vi "OMR_Automatic_Report_Generation .vi"() -> ()   [LabVIEW 2011]
uses:
  <vilib>/Utility/file.llb/Write To Spreadsheet File (string).vi
  <vilib>/vision/NI_Vision_Development_Module.lvlib
panel:
  out "Result":string[](array[string])
  in  "?":bool
  in  "Tab Control":T1(tab)
  out "Score":dbl
  out "Image 2":T2(plugin-control)
  in  "File Path":path
  out "File Path 2":string
  in  "Marks for\nCorrect Answe":dbl format="%#_6p"
  in  "6 to 10":string[](array[string])
  in  "1 to 5":string[](array[string])
  in  "16 to  20":string[](array[string])
  in  "11 to 15":string[](array[string])
  out "Score 2":dbl format="%_4f"
  out "0 to 5":dbl[](array[numeric])
  out "0 to 6":dbl[](array[numeric])
  out "0 to 7":dbl[](array[numeric])
  out "0 to 8":dbl[](array[numeric])
  out "Centroid (16 to 20)":cluster{"X Centroid":sgl, "Y Centroid":sgl} {"Y Centroid" format="%.2f"; "X Centroid" format="%.2f"}
  out "Centroid (1 to 5)":cluster{"X Centroid":sgl, "Y Centroid":sgl} {"Y Centroid" format="%.2f"; "X Centroid" format="%.2f"}
  out "Centroid (11 to 15)":cluster{"X Centroid":sgl, "Y Centroid":sgl} {"Y Centroid" format="%.2f"; "X Centroid" format="%.2f"}
  out "Centroid (6 to 10)":cluster{"X Centroid":sgl, "Y Centroid":sgl} {"Y Centroid" format="%.2f"; "X Centroid" format="%.2f"}
  out "1 to 5":string[](array[string])
  out "5 to 10":string[](array[string])
  out "11 to 15":string[](array[string])
  out "16 to 20":string[](array[string])
  out "1 to 6":dbl[](array[numeric])
  out "6 to 10":dbl[](array[numeric])
  out "11 to 16":dbl[](array[numeric])
  out "16 to 21":dbl[](array[numeric])
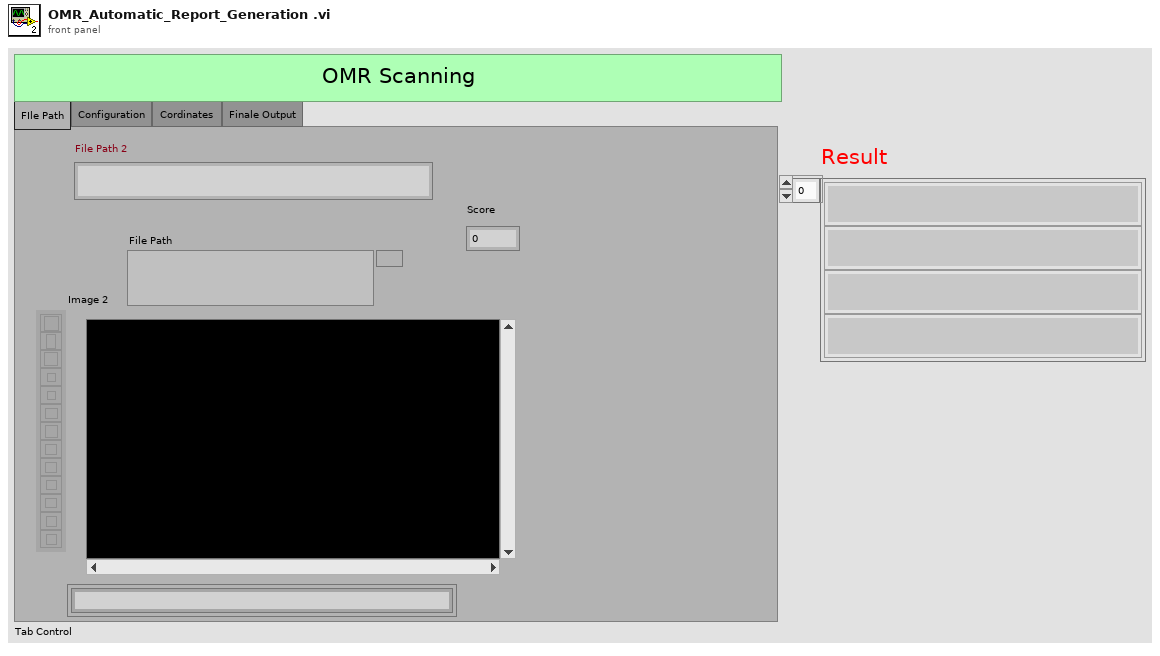
[diagram p1: front panel]
types:
  T1 = enum32{"FIle Path", "Configuration", "Cordinates ", "Finale Output"}
  T2 = typedef "IMAQ Image.ctl" = refnum<image>
  T3 = typedef "Image Type" = u32
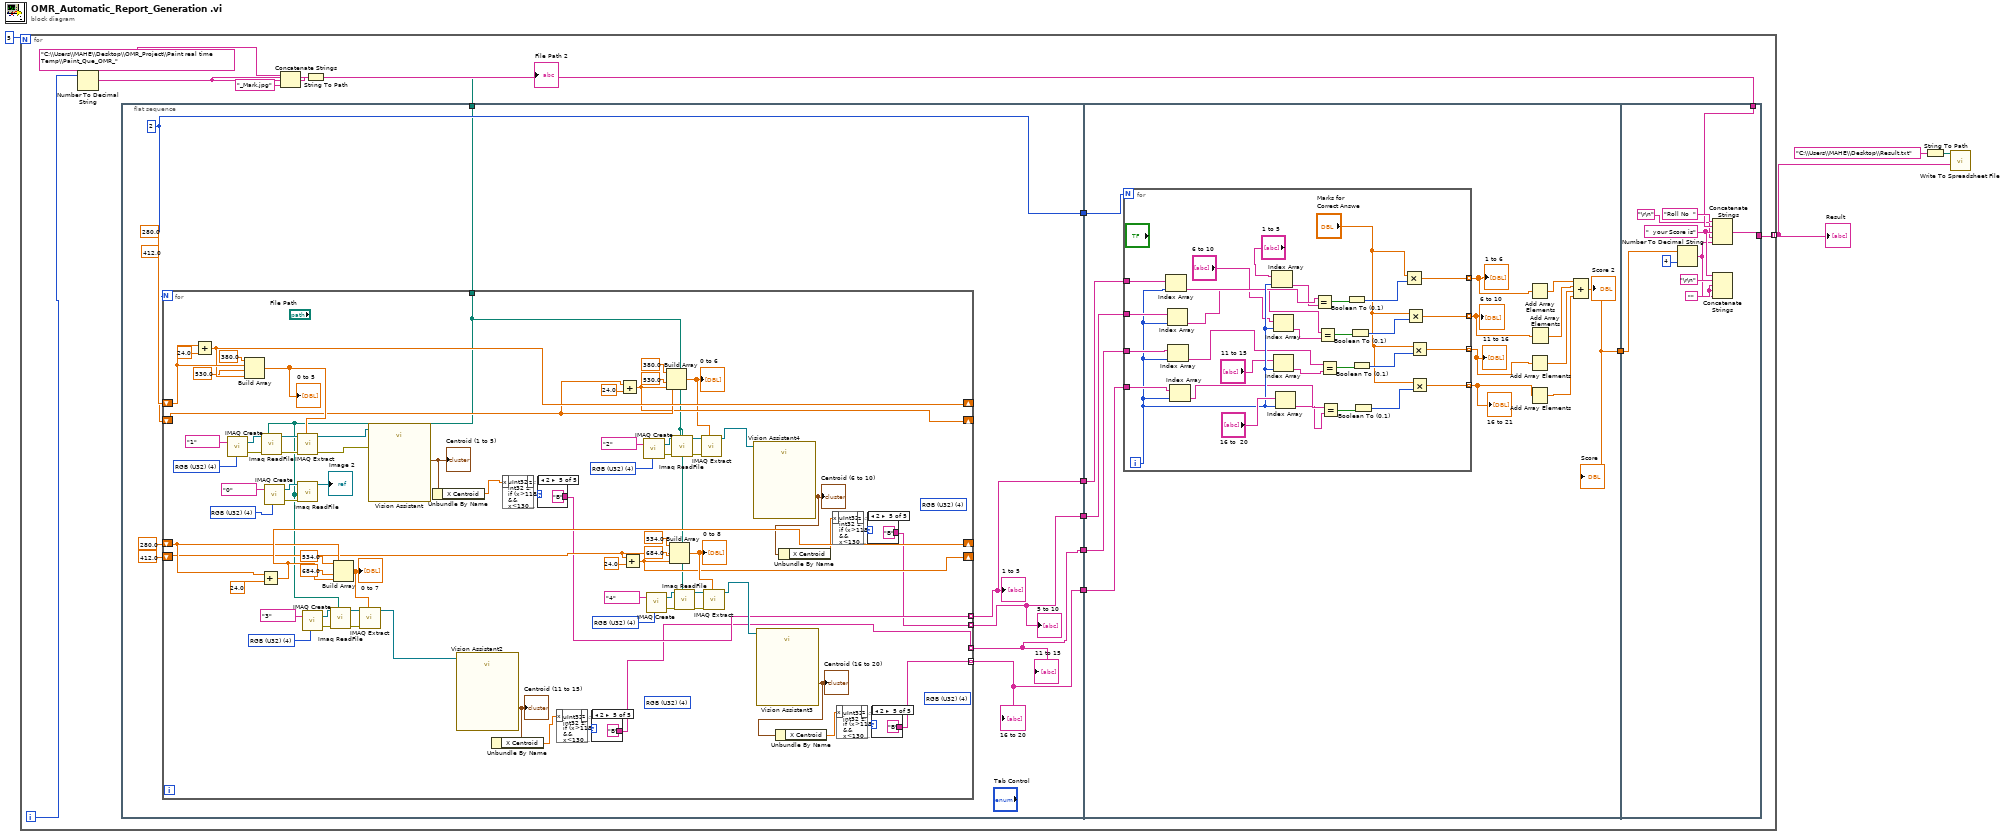
[diagram p0: block diagram]
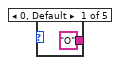
[diagram p2: hidden frame]
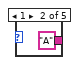
[diagram p3: hidden frame]
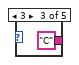
[diagram p4: hidden frame]
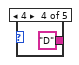
[diagram p5: hidden frame]
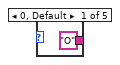
[diagram p6: hidden frame]
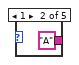
[diagram p7: hidden frame]
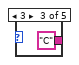
[diagram p8: hidden frame]
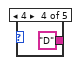
[diagram p9: hidden frame]
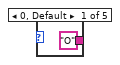
[diagram p10: hidden frame]
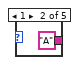
[diagram p11: hidden frame]
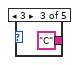
[diagram p12: hidden frame]
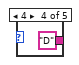
[diagram p13: hidden frame]
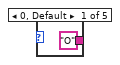
[diagram p14: hidden frame]
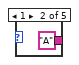
[diagram p15: hidden frame]
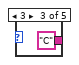
[diagram p16: hidden frame]
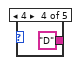
[diagram p17: hidden frame]
diagram:
  n1 = for {
    N: 5 -> [_]
    tunnel: [w5] -> w1 mode=indexing
    i -> [w9]
    n2 = Number To Decimal String(number=w9) -> (decimal integer string=w6:string)  [unwired: 1 in]
    n3 = flat-sequence {
      tunnel: [w23] -> w17
      tunnel: [w21] -> w16
      tunnel: [w22] -> w15
      tunnel: [w19] -> w14
      tunnel: [w20] -> w13
      tunnel: w8 -> [w18]
      tunnel: w17 -> [w135]
      tunnel: w16 -> [w134]
      tunnel: w15 -> [w132]
      tunnel: w14 -> [w133]
      tunnel: w13 -> [w136]
      tunnel: [w123] -> w12
      tunnel: w12 -> [w176]
      tunnel: w6 -> [w171]
      tunnel: [w167] -> w5
      frame #0 {
        w20 = 2
        n4 = for {
          N: w20 -> [_]
          shift-right: [w97] -> _
          shift-left: 280.0 -> [w98]
          shift-right: [w74] -> _
          shift-left: 412.0 -> [w75]
          shift-right: [w52] -> _
          shift-left: 280.0 -> [w50]
          shift-right: [w51] -> _
          shift-left: 412.0 -> [w49]
          tunnel: [w32] -> w23 mode=indexing
          tunnel: [w31] -> w21 mode=indexing
          tunnel: [w30] -> w19 mode=indexing
          tunnel: [w29] -> w22 mode=indexing
          tunnel: w18 -> [w28]
          (unwired) T3 4 items=["Grayscale (U8)", "Grayscale (I16)", "Grayscale (SGL)", "Complex (CSG)", "RGB (U32)", "HSL (U32)", "RGB (U64)"] ("Image Type")
          (unwired) T3 4 items=["Grayscale (U8)", "Grayscale (I16)", "Grayscale (SGL)", "Complex (CSG)", "RGB (U32)", "HSL (U32)", "RGB (U64)"] ("Image Type")
          (unwired) T3 4 items=["Grayscale (U8)", "Grayscale (I16)", "Grayscale (SGL)", "Complex (CSG)", "RGB (U32)", "HSL (U32)", "RGB (U64)"] ("Image Type")
          w59 = T3 4 items=["Grayscale (U8)", "Grayscale (I16)", "Grayscale (SGL)", "Complex (CSG)", "RGB (U32)", "HSL (U32)", "RGB (U64)"] ("Image Type")
          w66 = T3 4 items=["Grayscale (U8)", "Grayscale (I16)", "Grayscale (SGL)", "Complex (CSG)", "RGB (U32)", "HSL (U32)", "RGB (U64)"] ("Image Type")
          w81 = T3 4 items=["Grayscale (U8)", "Grayscale (I16)", "Grayscale (SGL)", "Complex (CSG)", "RGB (U32)", "HSL (U32)", "RGB (U64)"] ("Image Type")
          w92 = T3 4 items=["Grayscale (U8)", "Grayscale (I16)", "Grayscale (SGL)", "Complex (CSG)", "RGB (U32)", "HSL (U32)", "RGB (U64)"] ("Image Type")
          w95 = T3 4 items=["Grayscale (U8)", "Grayscale (I16)", "Grayscale (SGL)", "Complex (CSG)", "RGB (U32)", "HSL (U32)", "RGB (U64)"] ("Image Type")
          n5 = Add(x=w98, y=24.0) -> (x+y=w97:dbl)
          n6 = call "IMAQ Create"("Image Name"="1", "Image Type"=w95) -> ("New Image"=w99:T2, "error out"=w90:errorcluster)  [unwired: 2 in, 1 out]
          n7 = Build Array(380.0 ("element"), w98, 530.0 ("element"), w97) -> (w86:dbl[])
          "0 to 5" <- w86
          n8 = Add(x=w50, y=24.0) -> (x+y=w52:dbl)
          n9 = call "Imaq ReadFile"("File Path"=w28, "error in (no error)"=w90, "Image"=w99) -> ("error out"=w89:errorcluster, "Image Out"=w91:T2)  [unwired: 2 in, 5 out]
          n10 = call "IMAQ Create"("Image Name"="0", "Image Type"=w92) -> ("New Image"=w93:T2, "error out"=w85:errorcluster)  [unwired: 2 in, 1 out]
          n11 = call "IMAQ Extract"("Optional Rectangle"=w86, "error in (no error)"=w89, "Image Src"=w91) -> ("error out"=w88:errorcluster, "Image Dst Out"=w87:T2)  [unwired: 7 in]
          n12 = call "Imaq ReadFile"("File Path"=w28, "error in (no error)"=w85, "Image"=w93) -> ("Image Out"=→"Image 2":T2)  [unwired: 2 in, 6 out]
          n13 = call "IMAQ Create"("Image Name"="3", "Image Type"=w66) -> ("New Image"=w67:T2, "error out"=w64:errorcluster)  [unwired: 2 in, 1 out]
          n14 = call "Imaq ReadFile"("File Path"=w28, "error in (no error)"=w64, "Image"=w67) -> ("error out"=w63:errorcluster, "Image Out"=w65:T2)  [unwired: 2 in, 5 out]
          n15 = Build Array(534.0 ("element"), w50, 684.0 ("element"), w52) -> (w72:dbl[])
          "0 to 7" <- w72
          n16 = call "IMAQ Extract"("Optional Rectangle"=w72, "error in (no error)"=w63, "Image Src"=w65) -> ("Image Dst Out"=w47:T2)  [unwired: 7 in, 1 out]
          n17 = call "Vision Assistant"("Image In"=w87, "error in"=w88) -> ("Centroid (Centroid 1)"=w40:cluster{"X Centroid":sgl, "Y Centroid":sgl})  [unwired: 22 in, 3 out]
          "Centroid (1 to 5)" <- w40
          n18 = Unbundle By Name(w40) -> ("X Centroid"=w39:sgl)
          n19 = call "Vision Assistant2"("Image In"=w47) -> ("Centroid (Centroid 1)"=w34:cluster{"X Centroid":sgl, "Y Centroid":sgl})  [unwired: 23 in, 3 out]
          "Centroid (11 to 15)" <- w34
          n20 = Unbundle By Name(w34) -> ("X Centroid"=w33:sgl)
          n21 = formula code="uInt32 a;\nint32 z;\nif (x>118 && x<130)\nz=4;\n\nif (x>90 && x<103)\nz=3;\n\nif (x>40 && x<50)\nz=1;\n\nif (x>65 && x<75)\nz=2;"("x"=w39) -> ("z"=w44:i32)
          n22 = case shown="2" w44 {
            tunnel: ["O" "A" "C" "D" "B"] -> w32
            frame 0, Default {
            }
            frame 1 {
            }
            frame 3 {
            }
            frame 4 {
            }
            frame 2 {
            }
          }
          n23 = formula code="uInt32 a;\nint32 z;\nif (x>118 && x<130)\nz=4;\n\nif (x>90 && x<103)\nz=3;\n\nif (x>40 && x<50)\nz=1;\n\nif (x>65 && x<75)\nz=2;"("x"=w33) -> ("z"=w43:i32)
          n24 = case shown="2" w43 {
            tunnel: ["O" "A" "C" "D" "B"] -> w30
            frame 0, Default {
            }
            frame 1 {
            }
            frame 3 {
            }
            frame 4 {
            }
            frame 2 {
            }
          }
          n25 = Add(x=w75, y=24.0) -> (x+y=w74:dbl)
          n26 = Add(x=w49, y=24.0) -> (x+y=w51:dbl)
          n27 = call "IMAQ Create"("Image Name"="2", "Image Type"=w81) -> ("New Image"=w80:T2, "error out"=w83:errorcluster)  [unwired: 2 in, 1 out]
          n28 = call "IMAQ Create"("Image Name"="4", "Image Type"=w59) -> ("New Image"=w58:T2, "error out"=w61:errorcluster)  [unwired: 2 in, 1 out]
          n29 = Build Array(380.0 ("element"), w75, 530.0 ("element"), w74) -> (w73:dbl[])
          "0 to 6" <- w73
          n30 = Build Array(534.0 ("element"), w49, 684.0 ("element"), w51) -> (w53:dbl[])
          "0 to 8" <- w53
          n31 = call "Imaq ReadFile"("File Path"=w28, "error in (no error)"=w83, "Image"=w80) -> ("error out"=w84:errorcluster, "Image Out"=w82:T2)  [unwired: 2 in, 5 out]
          n32 = call "Imaq ReadFile"("File Path"=w28, "error in (no error)"=w61, "Image"=w58) -> ("error out"=w62:errorcluster, "Image Out"=w60:T2)  [unwired: 2 in, 5 out]
          n33 = call "IMAQ Extract"("Optional Rectangle"=w73, "error in (no error)"=w84, "Image Src"=w82) -> ("Image Dst Out"=w46:T2)  [unwired: 7 in, 1 out]
          n34 = call "IMAQ Extract"("Optional Rectangle"=w53, "error in (no error)"=w62, "Image Src"=w60) -> ("Image Dst Out"=w45:T2)  [unwired: 7 in, 1 out]
          n35 = call "Vision Assistant4"("Image In"=w46) -> ("Centroid (Centroid 1)"=w35:cluster{"X Centroid":sgl, "Y Centroid":sgl})  [unwired: 23 in, 3 out]
          "Centroid (6 to 10)" <- w35
          n36 = call "Vision Assistant3"("Image In"=w45) -> ("Centroid (Centroid 1)"=w38:cluster{"X Centroid":sgl, "Y Centroid":sgl})  [unwired: 23 in, 3 out]
          "Centroid (16 to 20)" <- w38
          n37 = Unbundle By Name(w38) -> ("X Centroid"=w37:sgl)
          n38 = Unbundle By Name(w35) -> ("X Centroid"=w36:sgl)
          n39 = formula code="uInt32 a;\nint32 z;\nif (x>118 && x<130)\nz=4;\n\nif (x>90 && x<103)\nz=3;\n\nif (x>40 && x<50)\nz=1;\n\nif (x>65 && x<75)\nz=2;"("x"=w36) -> ("z"=w41:i32)
          n40 = formula code="uInt32 a;\nint32 z;\nif (x>118 && x<130)\nz=4;\n\nif (x>90 && x<103)\nz=3;\n\nif (x>40 && x<50)\nz=1;\n\nif (x>65 && x<75)\nz=2;"("x"=w37) -> ("z"=w42:i32)
          n41 = case shown="2" w41 {
            tunnel: ["O" "A" "C" "D" "B"] -> w31
            frame 0, Default {
            }
            frame 1 {
            }
            frame 3 {
            }
            frame 4 {
            }
            frame 2 {
            }
          }
          n42 = case shown="2" w42 {
            tunnel: ["O" "A" "C" "D" "B"] -> w29
            frame 0, Default {
            }
            frame 1 {
            }
            frame 3 {
            }
            frame 4 {
            }
            frame 2 {
            }
          }
        }
        "1 to 5" <- w23
        "5 to 10" <- w21
        "11 to 15" <- w19
        "16 to 20" <- w22
      }
      frame #1 {
        n43 = for {
          N: w136 -> [_]
          tunnel: w135 -> [w166]
          tunnel: w134 -> [w165]
          tunnel: w133 -> [w164]
          tunnel: w132 -> [w163]
          tunnel: [w144] -> w128 mode=indexing
          tunnel: [w143] -> w129 mode=indexing
          tunnel: [w142] -> w131 mode=indexing
          tunnel: [w141] -> w130 mode=indexing
          i -> [w161]
          n44 = Index Array(array=w166, index=w161) -> (element=w160:string)
          n45 = Index Array(array=w165, index=w161) -> (element=w150:string)
          n46 = Index Array(array=w164, index=w161) -> (element=w151:string)
          n47 = Index Array(array=w163, index=w161) -> (element=w154:string)
          n48 = Index Array(array="1 to 5", index=w161) -> (element=w159:string)
          n49 = Index Array(array="6 to 10", index=w161) -> (element=w149:string)
          n50 = Index Array(array="11 to 15", index=w161) -> (element=w152:string)
          n51 = Index Array(array="16 to  20", index=w161) -> (element=w153:string)
          n52 = Equal?(x=w160, y=w159) -> (x = y?=w158:bool)
          n53 = Equal?(x=w150, y=w149) -> (x = y?=w157:bool)
          n54 = Equal?(x=w151, y=w152) -> (x = y?=w156:bool)
          n55 = Equal?(x=w154, y=w153) -> (x = y?=w155:bool)
          n56 = Boolean To (0,1)(Boolean=w158) -> (0, 1=w148:i16)
          n57 = Boolean To (0,1)(Boolean=w157) -> (0, 1=w146:i16)
          n58 = Boolean To (0,1)(Boolean=w156) -> (0, 1=w145:i16)
          n59 = Boolean To (0,1)(Boolean=w155) -> (0, 1=w147:i16)
          n60 = Multiply(x="Marks for\nCorrect Answe", y=w148) -> (x*y=w144:dbl)
          n61 = Multiply(x="Marks for\nCorrect Answe", y=w146) -> (x*y=w143:dbl)
          n62 = Multiply(x="Marks for\nCorrect Answe", y=w145) -> (x*y=w141:dbl)
          n63 = Multiply(x="Marks for\nCorrect Answe", y=w147) -> (x*y=w142:dbl)
        }
        "1 to 6" <- w128
        "6 to 10" <- w129
        "11 to 16" <- w130
        "16 to 21" <- w131
        n64 = Add Array Elements(numeric array=w128) -> (sum=w127:dbl)
        n65 = Add Array Elements(numeric array=w130) -> (sum=w125:dbl)
        n66 = Add Array Elements(numeric array=w131) -> (sum=w124:dbl)
        n67 = Add Array Elements(numeric array=w129) -> (sum=w126:dbl)
        n68 = Compound Arithmetic op=ADD(w127, w126, w125, w124) -> (w123:dbl)
        "Score 2" <- w123
        "Score" <- w123
      }
      frame #2 {
        w174 = ""
        w170 = "  your Score is"
        n69 = Number To Decimal String(number=w176, width (-)=i16 4) -> (decimal integer string=w168:string)
        n70 = Concatenate Strings("Roll No  " ("string"), w171, w170, "\r\n", w168) -> (w167:string)
        n71 = Concatenate Strings(w170, "\r\n", w174, w174, w168) -> ()  [unwired: 1 out]
      }
    }
    n72 = Concatenate Strings("C:\\Users\\MAHE\\Desktop\\OMR_Project\\Paint real time Temp\\Paint_Que_OMR_", w6, "_Mark.jpg" ("string")) -> (w11:string)
    "File Path 2" <- w11
    n73 = String To Path(string=w11) -> (path=w8:path)
  }
  "Result" <- w1
  n74 = String To Path(string="C:\\Users\\MAHE\\Desktop\\Result.txt") -> (path=w3:path)
  n75 = call-poly <vilib>:"Write To Spreadsheet File.vi"("1D data"=w1, "file path (dialog if empty)"=w3) -> ()  [unwired: 6 in, 1 out]
